vi "Build Current Sense Section.vi"(6 "Cancelled?":bool, 8 "error in (no error)":errorcluster, 9 "Card Position in":T1 {"Slot #" max=15}, 10 "Name in":string, 11 "Node Ptr in":u64) -> (0 "error out":errorcluster)   [LabVIEW 2014, in "SLSC configuration System Explorer.lvlib"]
uses:
  SLSC configuration System Explorer.lvlib
  Type Defs/Card Position.ctl
  Shared/SPI Utility/Slot #.ctl
  <vilib>/NI Veristand/Custom Device API/Custom Device Channel.ctl
  <vilib>/NI Veristand/Custom Device API/Custom Device Channel Type.ctl
  Shared/Constants.vi
  <vilib>/NI Veristand/Custom Device API/Custom Device API.lvlib
  Shared/SLSC configuration Shared.lvlib
  <vilib>/NI Veristand/Custom Device Tools/Custom Device Utility Library/Custom Device Utility Library.lvlib
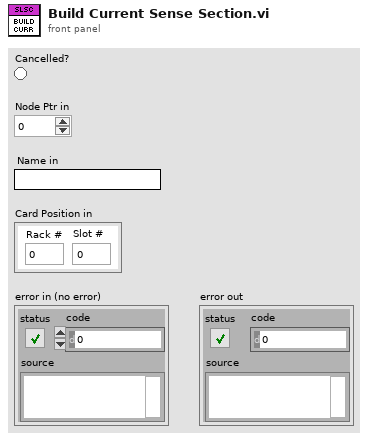
[diagram p1: front panel]
types:
  T1 = typedef "SLSC configuration Shared.lvlib/Card Position.ctl" = cluster{"Rack #":u8, "Slot #":T2}
  T2 = typedef "SLSC configuration Shared.lvlib/Slot #.ctl" = u8
  T3 = typedef "Custom Device API.lvlib/Custom Device Channel Type.ctl" = enum16{"Input", "Output"}
  T4 = typedef "Custom Device API.lvlib/Custom Device Channel.ctl" = cluster{"Type":T3, "Units":string, "Default Value":dbl, "Faultable":bool, "Scalable":bool}
  T5 = typedef "Custom Device API.lvlib/Custom Device Item Ref.ctl" = u64
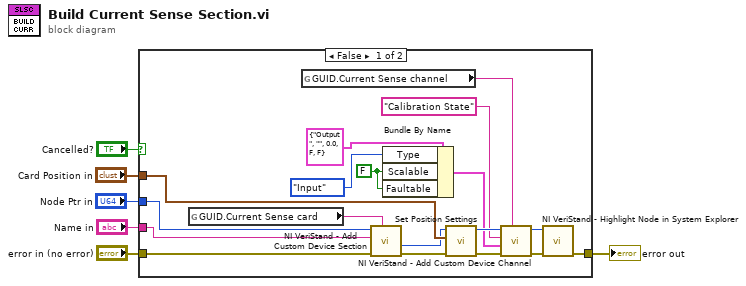
[diagram p0: block diagram]
diagram:
  n1 = case shown="False" "Cancelled?" {
    tunnel: "error in (no error)" -> [w24 w25]
    tunnel: "Node Ptr in" -> [w23 _]
    tunnel: "Card Position in" -> [w20 _]
    tunnel: [w15 w25] -> w5
    tunnel: "Name in" -> [w14 _]
    frame False {
      w10 = FALSE ("Scalable")
      n2 = global read "Constants.vi" "GUID.Current Sense card"() -> (w22:string)
      n3 = global read "Constants.vi" "GUID.Current Sense channel"() -> (w9:string)
      n4 = call <vilib>:"NI VeriStand - Add Custom Device Section.vi"("GUID (Default Section)"=w22, "error in (no error)"=w24, "Section Name"=w14, "Parent Ref in"=w23) -> ("error out"=w21:errorcluster, "Section Ptr"=w19:T5)  [unwired: 4 in, 2 out]
      n5 = Bundle By Name(cluster=T4 {"Type"=enum."Output", "Units"="", "Default Value"=0.0, "Faultable"=FALSE, "Scalable"=FALSE} ("Channel"), "Type"=Custom_Device_Channel_Type."Input", "Scalable"=w10, "Faultable"=w10) -> (w12:T4)
      n6 = call "Set Position Settings.vi"("error in (no error)"=w21, "Card Position"=w20, "Item Ref in"=w19) -> ("error out"=w18:errorcluster, "Item Ref out"=w17:T5)  [unwired: 7 in]
      n7 = call <vilib>:"NI VeriStand - Add Custom Device Channel.vi"("GUID (Default Channel)"=w9, "error in (no error)"=w18, "Channel"=w12, "Channel Name"="Calibration State", "Parent Ref in"=w17) -> ("error out"=w7:errorcluster, "Parent Ref out"=w16:T5)  [unwired: 3 in, 2 out]
      n8 = call <vilib>:"NI VeriStand - Highlight Node in System Explorer.vi"("error in (no error)"=w7, "Item Ref in"=w16) -> ("error out"=w15:errorcluster)  [unwired: 8 in, 1 out]
    }
    frame True {
    }
  }
  "error out" <- w5
